vi "GET FactorPotencia.vi"(8 "error in (no error)":errorcluster) -> (0 "error out":errorcluster, 3 "FACTORDEPOTENCIA":dbl[](array[numeric]))   [LabVIEW 2020, in "DB Previtech.lvlib"]
uses:
  DB Previtech.lvlib
  <vilib>/drjdpowell/SQLite Library/SQL Connection/Open (path).vi
  <vilib>/drjdpowell/SQLite Library/SQL Connection/Open (string).vi
  <vilib>/AdvancedString/Path To Command Line String.vi
  <vilib>/drjdpowell/SQLite Library/SQL Connection/Execute SQL (1D DBL results).vi
  <vilib>/drjdpowell/SQLite Library/SQL Connection/Connection.lvclass
  <vilib>/drjdpowell/SQLite Library/SQLite.lvlib
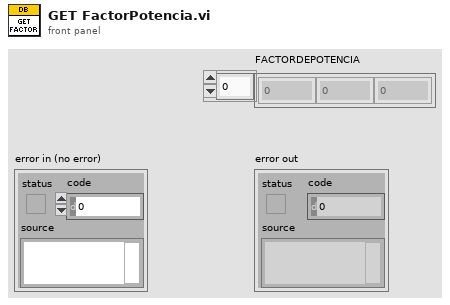
[diagram p1: front panel]
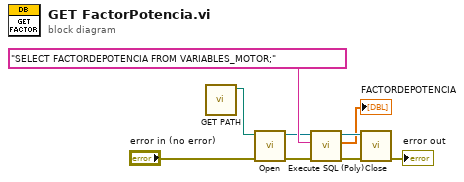
[diagram p0: block diagram]
diagram:
  n1 = call "GET PATH.vi"() -> ("DB Path"=w7:path)  [unwired: 11 in]
  n2 = call-poly <vilib>:"Open.vi"("error in (no error)"="error in (no error)", "db file"=w7) -> ("error out"=w4:errorcluster, "SQLite Connection"=w5:refnum<class "Connection.lvclass">)  [unwired: 8 in]
  n3 = call-poly <vilib>:"Execute SQL (Poly).vi"("error in (no error)"=w4, "SQL"="SELECT FACTORDEPOTENCIA FROM VARIABLES_MOTOR;", "SQLite Connection in"=w5) -> ("error out"=w2:errorcluster, "Result Set"=→"FACTORDEPOTENCIA":dbl[], "SQLite Connection"=w3:refnum<class "Connection.lvclass">)  [unwired: 5 in, 1 out]
  n4 = call-dynamic "Close.vi"("error in (no error)"=w2, "SQLite Connection in"=w3) -> ("error out"=→"error out":errorcluster)  [unwired: 9 in]
